vi "SCREEN_1.vi"(8 "error in (no error)":errorcluster, 11 "Main_Data_Flow":T1={"Hardware Setting"=path "", "Hardware"={"Monitor Primary 1"=1, "Monitor 2"=2, "Monitor 3"=3, "Scanner IP"="", "Scanner 2"="", "Scanner 3"="", "Printer IP"="", "Printer 2"="", "Printer 3"=""}, "SOP Path"=path "", "PNR Path"=path "", "PRN Data"=""}) -> (0 "error OUT":errorcluster)   [LabVIEW 2017]
doc: "Use this template to build a user interface event handler design pattern. Use this pattern for dialog boxes and other user interfaces. You also can create and execute user-defined events that the VI can handle the same way as user interface events."
uses:
  Controls/Main_Loop_Data_Flow.ctl
  Controls/PLC_DATA_READ.ctl
  Controls/PLC_DATA_WRITE.ctl
  Controls/AUTO_STATE_QUEUE.ctl
  Controls/Screen1_st.ctl
  <vilib>/Utility/error.llb/DialogType.ctl
  <userlib>/_OpenG.lib/array/array.llb/Sort 1D Array (I32)__ogtk.vi
  <vilib>/Utility/config.llb/Read Key (U32).vi
  <vilib>/Utility/config.llb/NI_LVConfig.lvlib
panel:
  out "Scanner Status":bool
  out "Scanned data":string
  out "Stop scanner":bool
  out "date/time string":string
  out "Varient Running":string
  out "Error Status in PLC Loop":errorcluster
  out "DATE/TIME":string
  out "Machine Name":string
  out "Weight":i32 format="%.0f gm"
  out "Cycle Result":bool
  out "Dispaly No.":string
  out "PLC to Labview Data":i32[](array[numeric])
  out "Cycle Status":string
  out "Scan Code":string
  out "sop picture":picture
  in  "Close":bool
  # "Resolution: 1920 x 1080 pixels"
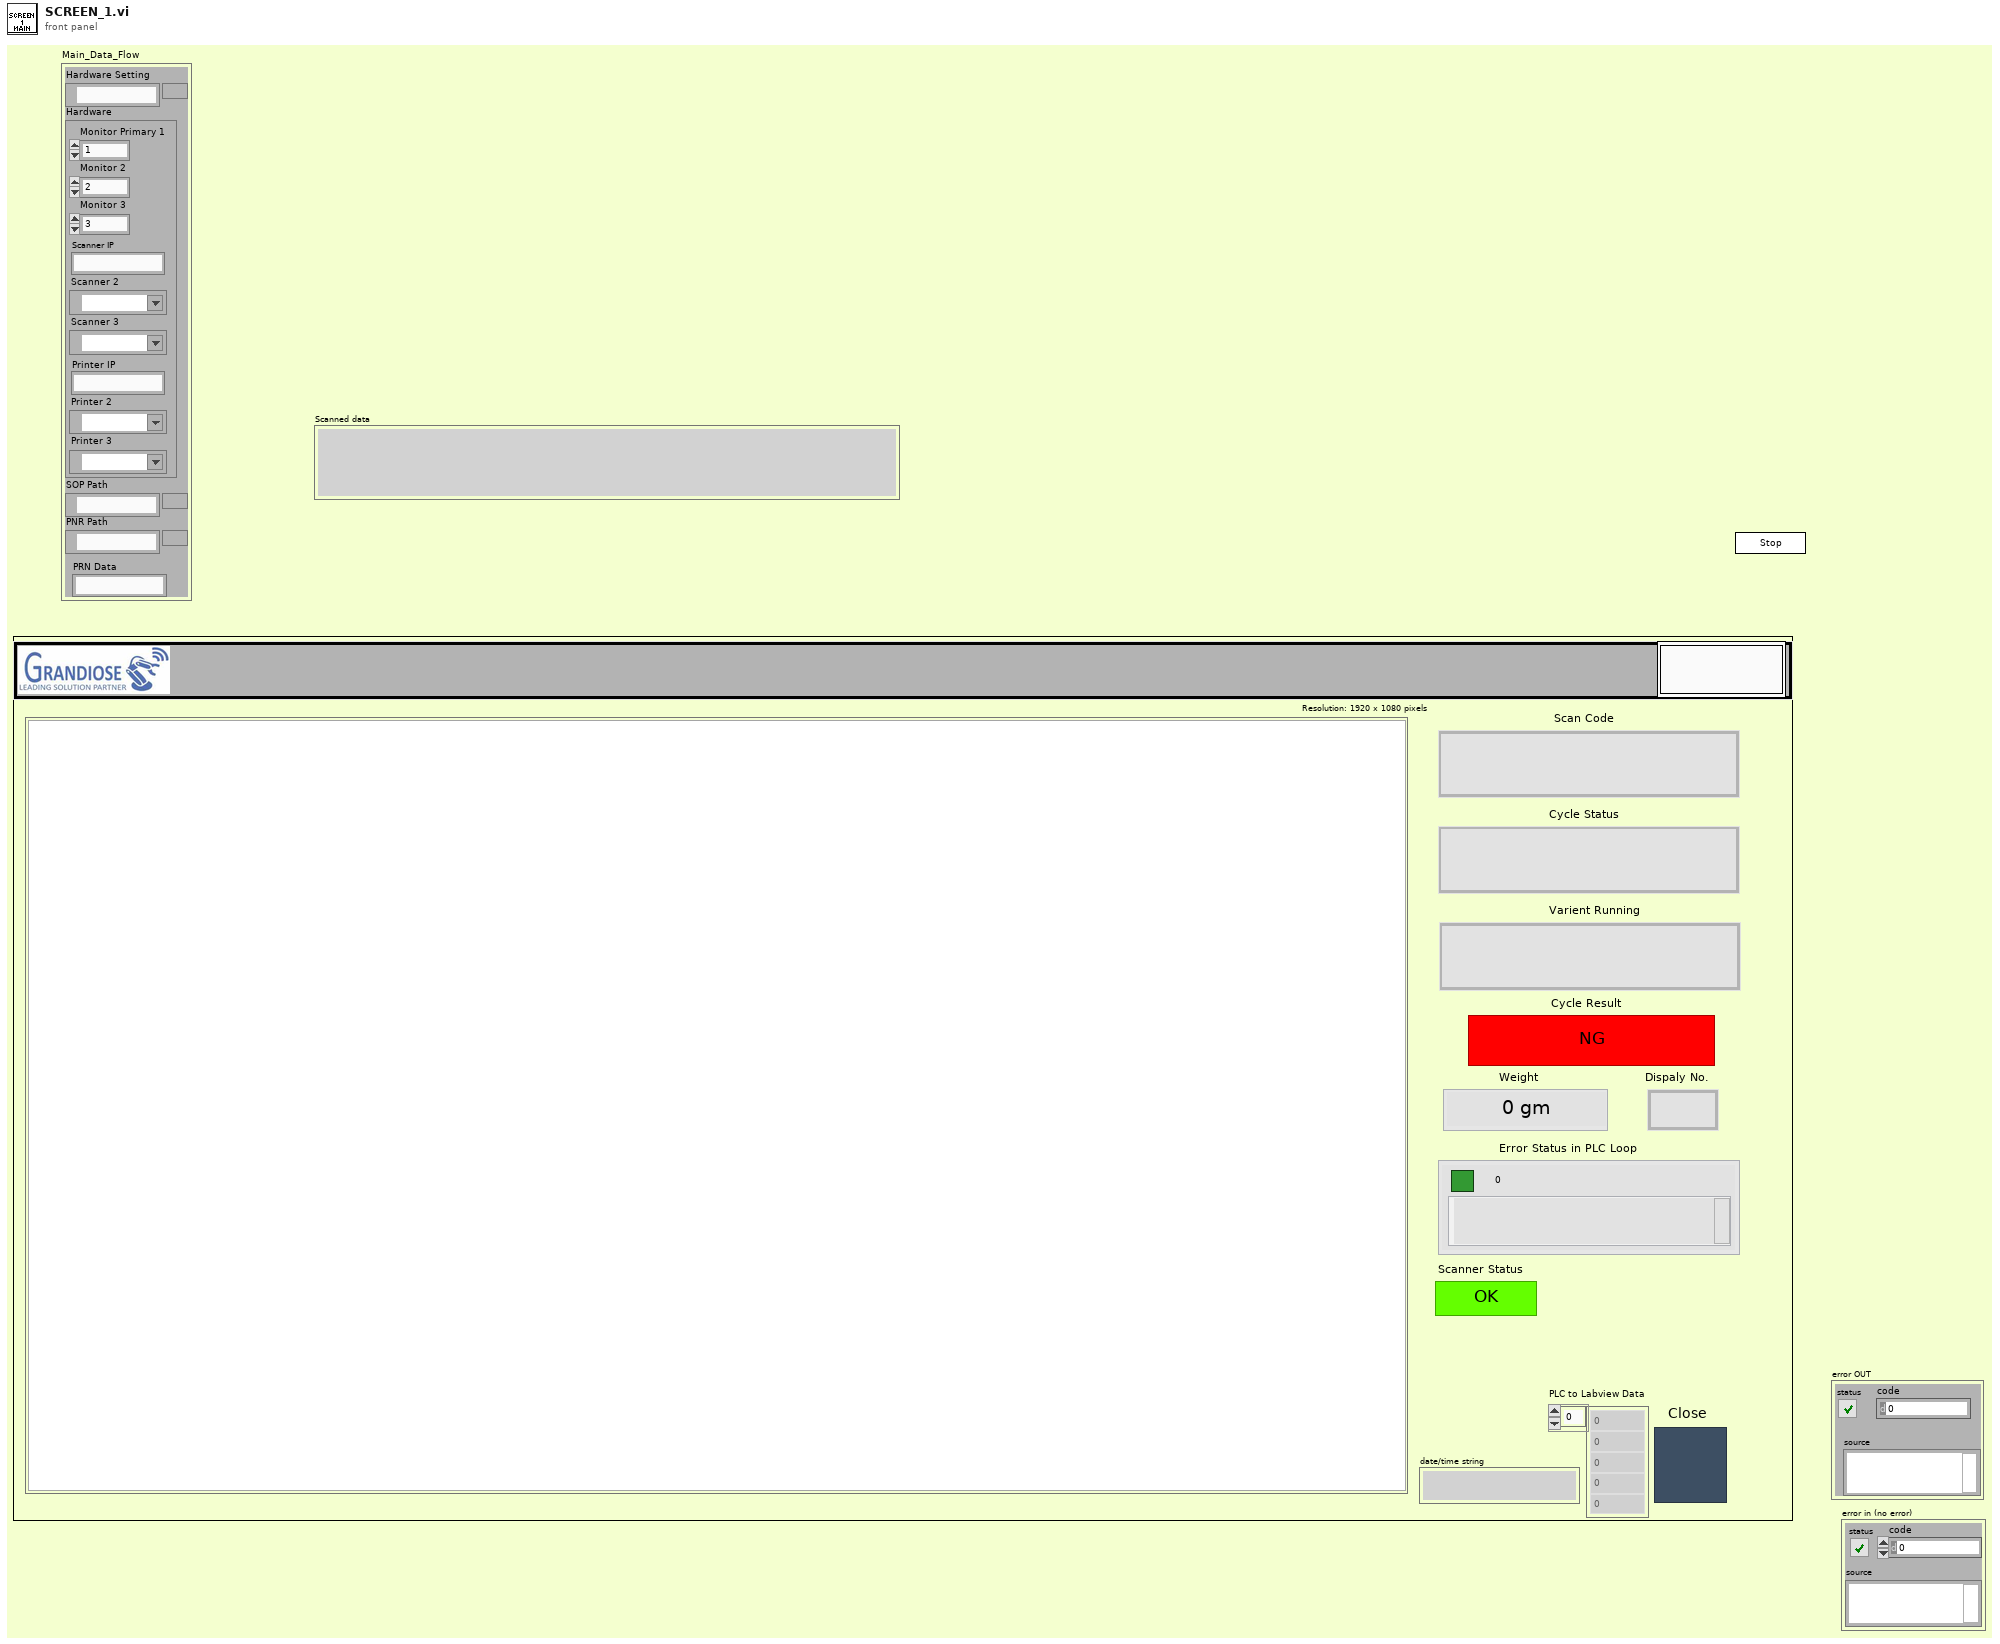
[diagram p1: front panel]
types:
  T1 = typedef "Main_Loop_Data_Flow.ctl" = cluster{"Hardware Setting":path, "Hardware":cluster{"Monitor Primary 1":u16, "Monitor 2":u16, "Monitor 3":u16, "Scanner IP":string, "Scanner 2":refnum<visa-resource-name>, "Scanner 3":refnum<visa-resource-name>, "Printer IP":string, "Printer 2":refnum<visa-resource-name>, "Printer 3":refnum<visa-resource-name>}, "SOP Path":path, "PNR Path":path, "PRN Data":string}
  T2 = typedef "AUTO_STATE_QUEUE.ctl" = enum16{"CREATE Q", "EN Q", "DE Q", "CLOSE Q"}
  T3 = typedef "PLC_DATA_READ.ctl" = cluster{"PLC to Labview Data":i32[], "Error Status in PLC Loop":errorcluster}
  T4 = cluster{"notifier out":refnum<notifier>, "SOP Path":path, "All Files SOP":path[], "PLC RCV data":T3, "Varient No.":u32[], "Varient name":string[], "Scanner IP":string, "Printer IP":string, "Printer ref":refnum<k5>, "PRN Data":string, "queue out":refnum<queue>}
  T5 = typedef "DialogType.ctl" = u16
  T6 = typedef "Screen1_st.ctl" = enum16{"Int", "Int2", "Wait", "Cluster_Update", "Cycle_Cmplt", "Varient_Updated", "Print_Code", "Error_Handling", "Exit"}
  T7 = typedef "imagedata.ctl" = cluster{"image type":i32, "image depth":i32, "image":u8[], "mask":u8[], "colors":u32[], "Rectangle":cluster{"left":i16, "top":i16, "right":i16, "bottom":i16}}
  T8 = typedef "PLC_DATA_WRITE.ctl" = cluster{"Register to write":u16, "Labview to PLC Data":u16}
  T9 = enum32{"invalid app kind", "Development System", "Run Time System", "Student Edition", "Embedded LabVIEW", "Evaluation", "Custom"}
  T10 = typedef "NI_LVConfig.lvlib/Config Data RefNum.ctl" = refnum<k1>
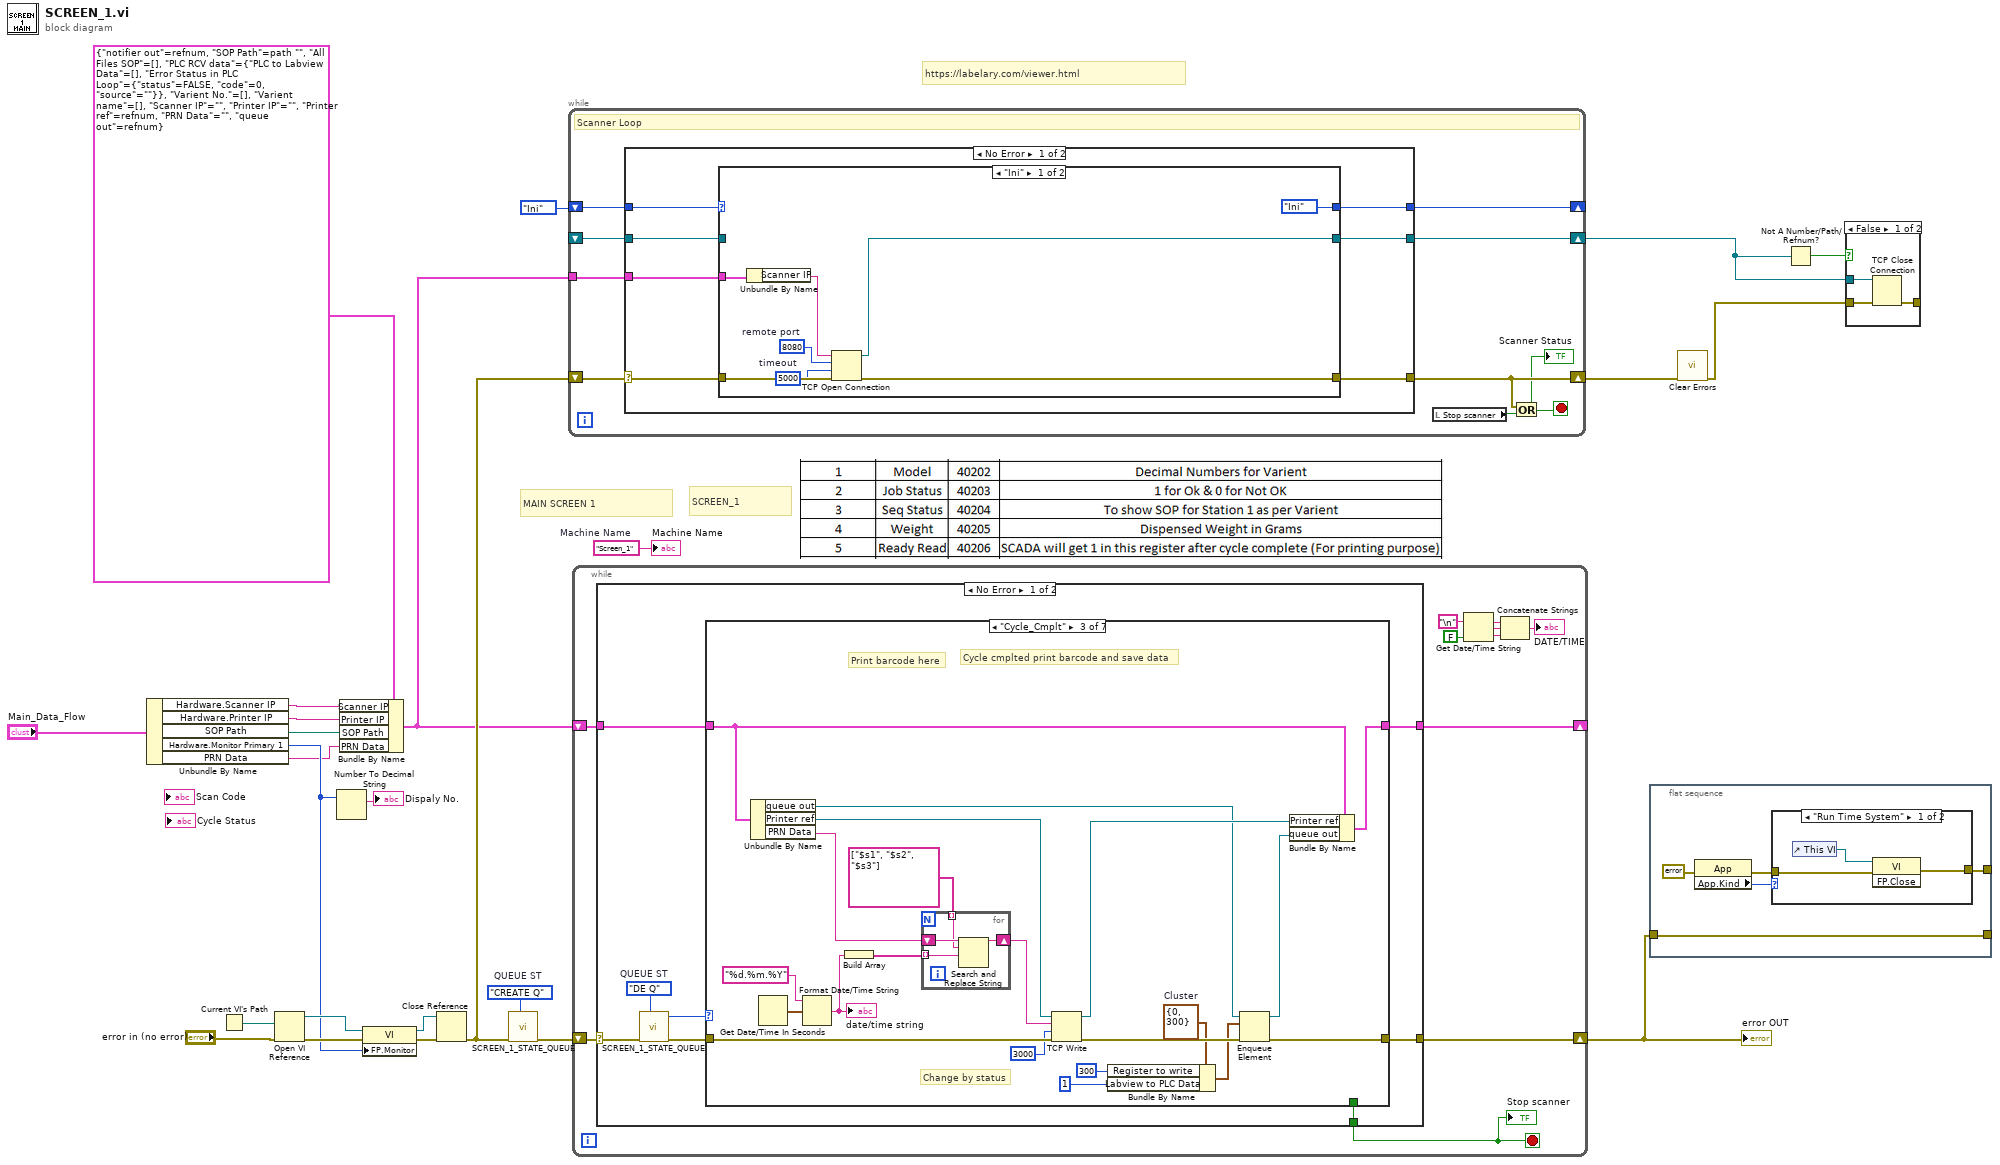
[diagram p0: block diagram]
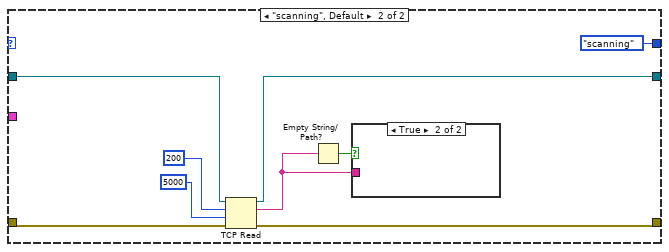
[diagram p3: hidden frame]
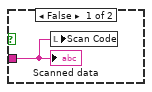
[diagram p4: hidden frame]
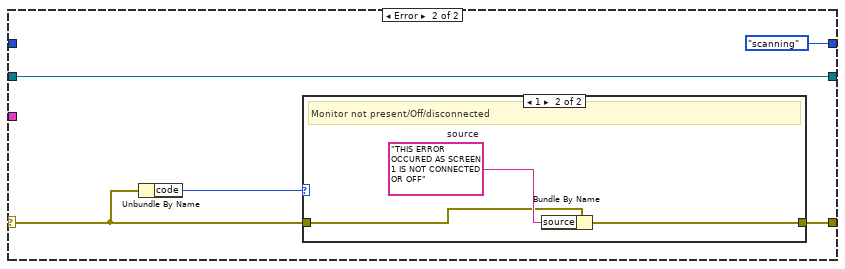
[diagram p5: hidden frame]
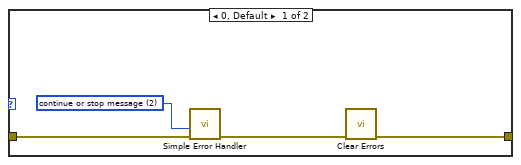
[diagram p6: hidden frame]
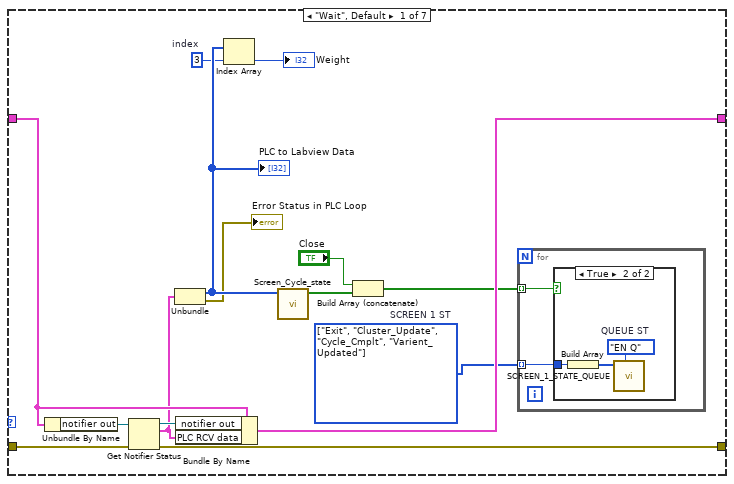
[diagram p8: hidden frame]
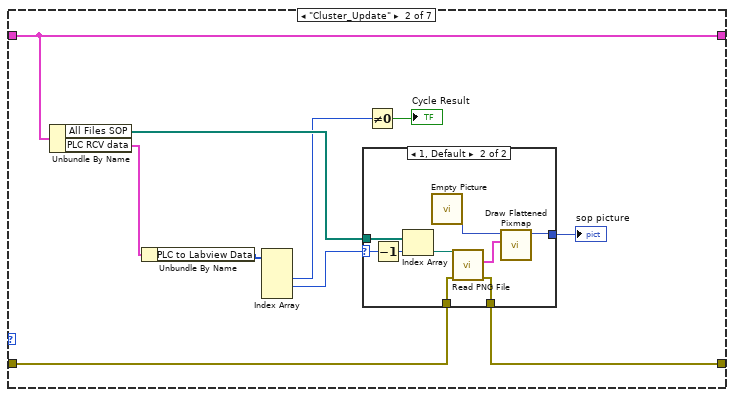
[diagram p10: hidden frame]
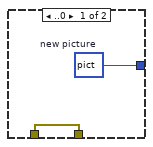
[diagram p11: hidden frame]
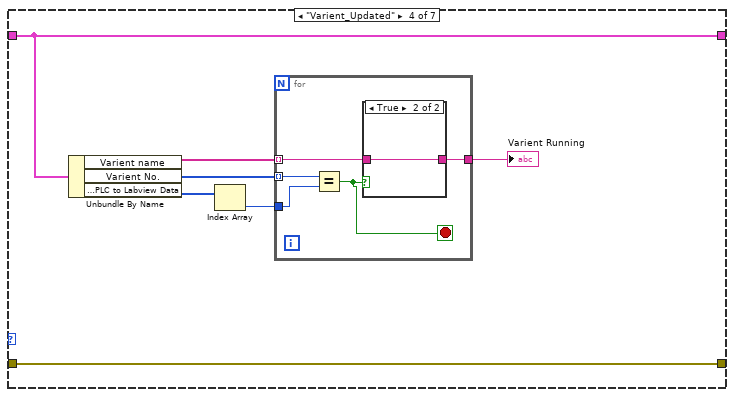
[diagram p12: hidden frame]
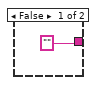
[diagram p13: hidden frame]
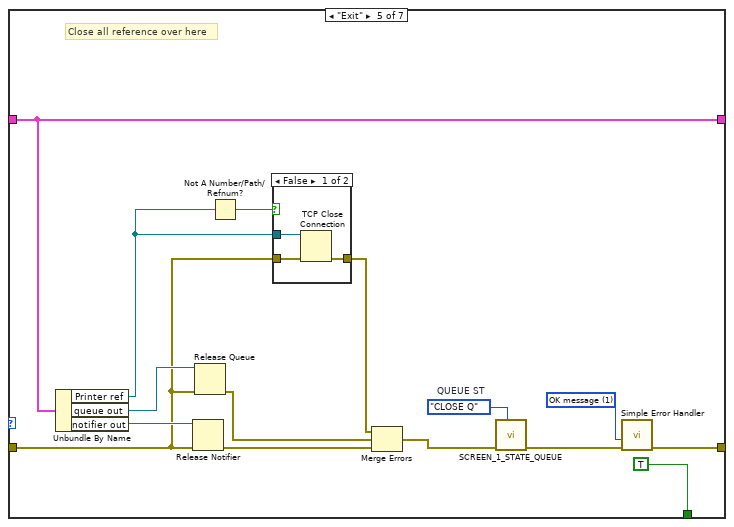
[diagram p14: hidden frame]
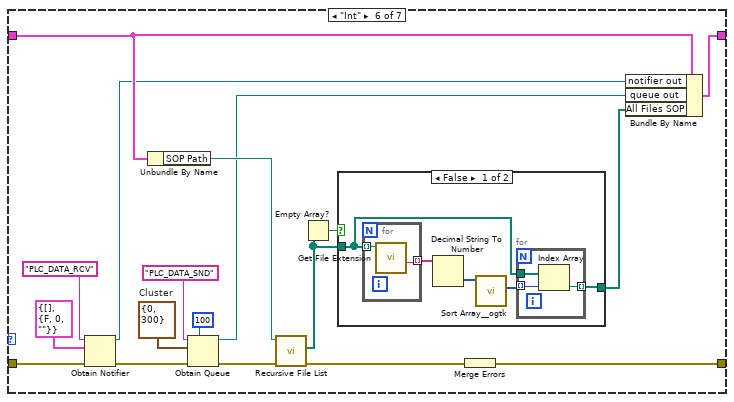
[diagram p16: hidden frame]
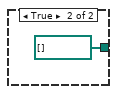
[diagram p17: hidden frame]
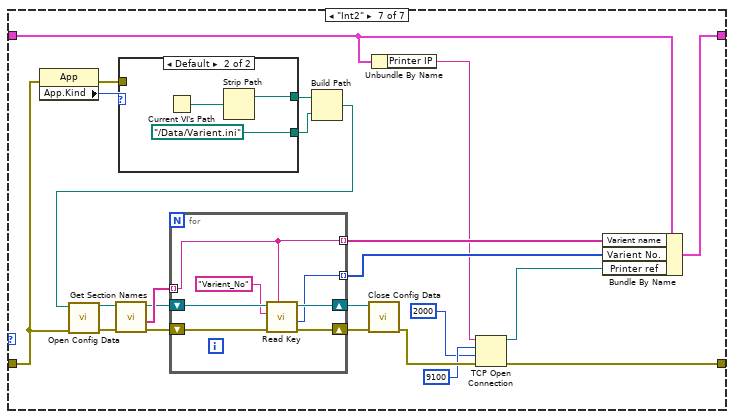
[diagram p18: hidden frame]
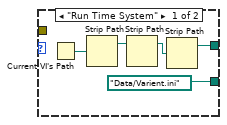
[diagram p19: hidden frame]
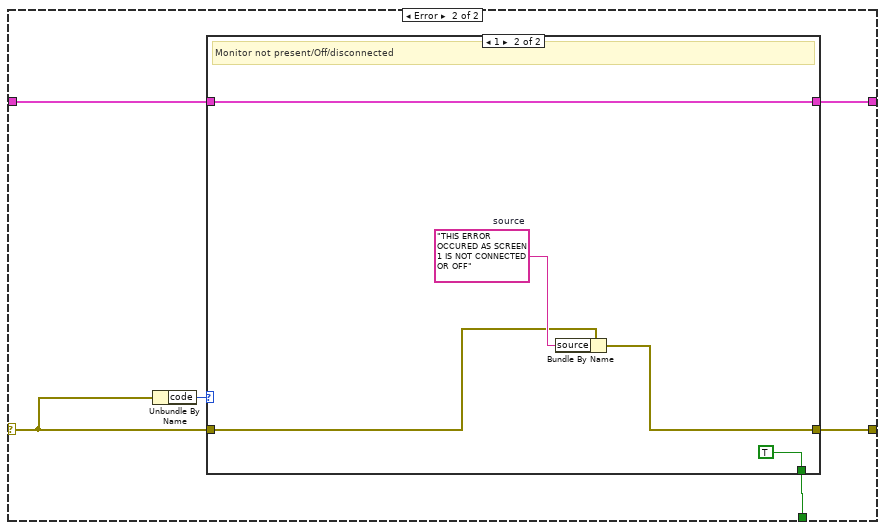
[diagram p20: hidden frame]
diagram:
  w10 = AUTO_STATE_QUEUE."CREATE Q"  # QUEUE ST
  w19 = "Screen_1"  # Machine Name
  # "https://labelary.com/viewer.html"
  # "MAIN SCREEN 1"
  # "SCREEN_1"
  n1 = Unbundle By Name("Main_Data_Flow") -> ("Hardware.Scanner IP"=w15:string, "Hardware.Printer IP"=w16:string, "SOP Path"=w9:path, "Hardware.Monitor Primary 1"=w12:u16, "PRN Data"=w8:string)
  n2 = Current VI's Path() -> (path=w25:path)
  n3 = Open VI Reference(vi path=w25, error in (no error)="error in (no error)") -> (vi reference=w21:refnum<vi>, error out=w22:errorcluster)  [unwired: 4 in]
  n4 = Number To Decimal String(number=w12) -> (decimal integer string=→"Dispaly No.":string)  [unwired: 1 in]
  n5 = Bundle By Name(cluster=T4 {"notifier out"=refnum, "SOP Path"=path "", "All Files SOP"=[], "PLC RCV data"={"PLC to Labview Data"=[], "Error Status in PLC Loop"={"status"=FALSE, "code"=0, "source"=""}}, "Varient No."=[], "Varient name"=[], "Scanner IP"="", "Printer IP"="", "Printer ref"=refnum, "PRN Data"="", "queue out"=refnum}, "Scanner IP"=w15, "Printer IP"=w16, "SOP Path"=w9, "PRN Data"=w8) -> (w5:T4)
  n6 = property class="VI"(reference=w21, error in=w22, "FP.Monitor"=w12) -> (reference out=w24:refnum<vi>, error out=w23:errorcluster)
  n7 = Close Reference(reference=w24, error in (no error)=w23) -> (error out=w7:errorcluster)
  n8 = call "SCREEN_1_STATE_QUEUE.vi"("QUEUE ST"=w10, "error in"=w7) -> ("error OUT"=w11:errorcluster)  [unwired: 8 in, 1 out]
  n9 = while {
    shift-right: [w32] -> w4
    shift-left: w7 -> [w34]
    shift-right: [w30] -> _
    shift-left: enum16{"Ini", "scanning", "Close"}."Ini" -> [w31]
    tunnel: w5 -> [w29]
    shift-right: [w28] -> w1
    shift-left: _ -> [w27]
    stop <- w26 stop-if-true
    # "Scanner Loop"
    n10 = case shown="No Error" w34 {
      selector: w34 -> [w41 w63]
      tunnel: [w40 w62] -> w32
      tunnel: w31 -> [w39 _]
      tunnel: [w38 enum16{"Ini", "scanning", "Close"}."scanning"] -> w30
      tunnel: w29 -> [w37 _]
      tunnel: [w36 w60] -> w28
      tunnel: w27 -> [w35 w60]
      frame No Error {
        n11 = case shown="\"Ini\"" w39 {
          tunnel: w41 -> [w47 w53]
          tunnel: [w46 w52] -> w40
          tunnel: [enum16{"Ini", "scanning", "Close"}."Ini" enum16{"Ini", "scanning", "Close"}."scanning"] -> w38
          tunnel: w37 -> [w48 _]
          tunnel: [w42 w50] -> w36
          tunnel: w35 -> [_ w51]
          frame "Ini" {
            w43 = 5000  # timeout
            w44 = u16 8080  # remote port
            n12 = Unbundle By Name(w48) -> ("Scanner IP"=w45:string)
            n13 = TCP Open Connection(address=w45, remote port or service name=w44, timeout ms (60000)=w43, error in (no error)=w47) -> (connection ID=w42:refnum<k5>, error out=w46:errorcluster)  [unwired: 1 in]
          }
          frame "scanning", Default {
            n14 = TCP Read(connection ID=w51, bytes to read=200, error in (no error)=w53, 9:5000 ("timeout ms (25000)")) -> (connection ID out=w50:refnum<k5>, data out=w56:string, error out=w52:errorcluster)  [unwired: 1 in]
            n15 = Empty String/Path?(string/path=w56) -> (empty?=w57:bool)
            n16 = case shown="True" w57 {
              tunnel: w56 -> [w59 _]
              frame False {
                n17 = local write "Scan Code"(w59) -> ()
                "Scanned data" <- w59
              }
              frame True {
              }
            }
          }
        }
      }
      frame Error {
        n18 = Unbundle By Name(w63) -> ("code"=w64:i32)
        n19 = case shown="1" w64 {
          tunnel: w63 -> [w68 w70]
          tunnel: [w66 w69] -> w62
          frame 0, Default {
            w65 = T5 2 items=["no dialog", "OK message", "continue or stop message", "OK message + warnings", "continue/stop + warnings"] ("type of dialog (OK msg:1)")
            n20 = call <vilib>:"Simple Error Handler.vi"("type of dialog (OK msg:1)"=w65, "error in (no error)"=w68) -> ("error out"=w67:errorcluster)  [unwired: 3 in, 4 out]
            n21 = call <vilib>:"Clear Errors.vi"("error in (no error)"=w67) -> ("error out"=w66:errorcluster)  [unwired: 5 in, 1 out]
          }
          frame 1 {
            w71 = "THIS ERROR OCCURED AS SCREEN 1 IS NOT CONNECTED OR OFF"  # source
            # "Monitor not present/Off/disconnected"
            n22 = Bundle By Name(cluster=w70, "source"=w71) -> (w69:errorcluster)
          }
        }
      }
    }
    n23 = local read "Stop scanner"() -> (w33:bool)
    n24 = Or(x=w32, y=w33) -> (x .or. y?=w26:bool)
    "Scanner Status" <- w26
  }
  n25 = while {
    shift-right: [w81] -> w14
    shift-left: w11 -> [w80]
    shift-right: [w78] -> _
    shift-left: w5 -> [w79]
    stop <- w72 stop-if-true
    n26 = case shown="No Error" w80 {
      selector: w80 -> [w86 w259]
      tunnel: [w82 w260] -> w72
      tunnel: [w89 w261] -> w81
      tunnel: w79 -> [w88 w257]
      tunnel: [w87 w256] -> w78
      frame No Error {
        w84 = AUTO_STATE_QUEUE."DE Q"  # QUEUE ST
        n27 = call "SCREEN_1_STATE_QUEUE.vi"("QUEUE ST"=w84, "error in"=w86) -> ("error OUT"=w85:errorcluster, "SCREEN 1"=w83:T6)  [unwired: 8 in]
        n28 = case shown="\"Cycle_Cmplt\"" w83 {
          tunnel: w85 -> [w104 w117 w151 w162 w172 w201 w229]
          tunnel: [w103 w116 w137 w162 w179 w206 w224] -> w89
          tunnel: w88 -> [w99 w119 w148 w161 w184 w205 w223]
          tunnel: [w100 w119 w147 w161 w184 w204 w228] -> w87
          tunnel: [_ _ _ _ TRUE _ _] -> w82
          frame "Wait", Default {
            w92 = 3  # index
            w95 = T6[] [enum."Exit", enum."Cluster_Update", enum."Cycle_Cmplt", enum."Varient_Updated"] items=["Int", "Int2", "Wait", "Cluster_Update", "Cycle_Cmplt", "Varient_Updated", "Print_Code", "Error_Handling", "Exit"]  # SCREEN 1 ST
            n29 = Unbundle By Name(w99) -> ("notifier out"=w102:refnum<notifier>)
            n30 = Get Notifier Status(notifier=w102, error in (no error)=w104) -> (notifier out=w101:refnum<notifier>, current notification=w91:T3, error out=w103:errorcluster)  [unwired: 2 out]
            n31 = Unbundle(w91) -> ("PLC to Labview Data"=w93:i32[], "Error Status in PLC Loop"=→"Error Status in PLC Loop":errorcluster)
            "PLC to Labview Data" <- w93
            n32 = Bundle By Name(cluster=w99, "notifier out"=w101, "PLC RCV data"=w91) -> (w100:T4)
            n33 = Index Array(array=w93, index=w92) -> (element=→"Weight":i32)
            n34 = call "Screen_Cycle_state.vi"("PLC to Labview Data"=w93) -> ("Cyc St"=w97:bool[])  [unwired: 10 in]
            n35 = Build Array (concatenate)("Close", w97) -> (w96:bool[])
            n36 = for {
              tunnel: w96 -> [w106] mode=indexing
              tunnel: w95 -> [w105] mode=indexing
              n37 = case shown="True" w106 {
                tunnel: w105 -> [_ w108]
                frame False {
                }
                frame True {
                  w109 = AUTO_STATE_QUEUE."EN Q"  # QUEUE ST
                  n38 = Build Array(w108) -> (w107:T6[])
                  n39 = call "SCREEN_1_STATE_QUEUE.vi"("QUEUE ST"=w109, "SCREEN 1 ST"=w107) -> ()  [unwired: 8 in, 2 out]
                }
              }
            }
          }
          frame "Cluster_Update" {
            n40 = Unbundle By Name(w119) -> ("All Files SOP"=w118:path[], "PLC RCV data"=w115:T3)
            n41 = Unbundle By Name(w115) -> ("PLC to Labview Data"=w114:i32[])
            n42 = Index Array(array=w114) -> (element #2=w111:i32, element #3=w113:i32)  [unwired: 4 in, 2 out]
            n43 = case shown="1, Default" w113 {
              selector: w113 -> [_ w124]
              tunnel: w118 -> [_ w127]
              tunnel: w117 -> [w121 w126]
              tunnel: [w121 w125] -> w116
              tunnel: [w120 w122] -> w110
              frame ..0 {
                w120 = picture data[5B]  # new picture
              }
              frame 1, Default {
                n44 = Decrement(x=w124) -> (x-1=w123:i32)
                n45 = Index Array(array=w127, index=w123) -> (element=w128:path)
                n46 = call "Empty Picture"() -> ("empty picture"=w129:picture)
                n47 = call <vilib>:"Read PNG File.vi"("error in (no error)"=w126, "path to PNG file"=w128) -> ("error out"=w125:errorcluster, "image data"=w130:T7)  [unwired: 7 in, 1 out]
                n48 = call <vilib>:"Draw Flattened Pixmap.vi"("image data"=w130, "picture"=w129) -> ("new picture"=w122:picture)  [unwired: 7 in]
              }
            }
            "sop picture" <- w110
            n49 = Not Equal To 0?(x=w111) -> (x != 0?=→"Cycle Result":bool)
          }
          frame "Cycle_Cmplt" {
            w134 = T8 {"Register to write"=0, "Labview to PLC Data"=300}  # Cluster
            # "Change by status"
            # "Print barcode here"
            # "Cycle cmplted print barcode and save data"
            n50 = Unbundle By Name(w148) -> ("queue out"=w136:refnum<queue>, "Printer ref"=w149:refnum<k5>, "PRN Data"=w141:string)
            n51 = Get Date/Time In Seconds() -> (seconds since 1Jan1904=w144:timestamp)
            n52 = Format Date/Time String(time format string (%c)="%d.%m.%Y", seconds (now)=w144) -> (date/time string=w139:string)  [unwired: 1 in]
            "date/time string" <- w139
            n53 = Build Array(w139) -> (w138:string[])
            n54 = for {
              shift-right: [w155] -> w140
              shift-left: w141 -> [w154]
              tunnel: string[] ["$s1", "$s2", "$s3"] -> [w153] mode=indexing
              tunnel: w138 -> [w152] mode=indexing
              n55 = Search and Replace String(input string=w154, search string=w153, replace string=w152) -> (result string=w155:string)  [unwired: 5 in, 3 out]
            }
            n56 = TCP Write(connection ID=w149, data in=w140, error in (no error)=w151, 9:3000 ("timeout ms (25000)")) -> (connection ID out=w146:refnum<k5>, error out=w150:errorcluster)  [unwired: 1 out]
            n57 = Bundle By Name(cluster=w134, "Register to write"=u16 300 ("timeout ms (25000)"), "Labview to PLC Data"=u16 1 ("timeout ms (25000)")) -> (w133:T8)
            n58 = Enqueue Element(queue=w136, element=w133, error in (no error)=w150) -> (queue out=w135:refnum<queue>, error out=w137:errorcluster)  [unwired: 1 in, 1 out]
            n59 = Bundle By Name(cluster=w148, "Printer ref"=w146, "queue out"=w135) -> (w147:T4)
          }
          frame "Varient_Updated" {
            n60 = Unbundle By Name(w161) -> ("Varient name"=w157:string[], "Varient No."=w159:u32[], "PLC RCV data.PLC to Labview Data"=w160:i32[])
            n61 = Index Array(array=w160) -> (element=w158:i32)  [unwired: 1 in]
            n62 = for {
              tunnel: w159 -> [w167] mode=indexing
              tunnel: w158 -> [w166]
              tunnel: [w165] -> w156
              tunnel: w157 -> [w164] mode=indexing
              stop <- w163 stop-if-true
              n63 = Equal?(x=w167, y=w166) -> (x = y?=w163:bool)
              n64 = case shown="True" w163 {
                tunnel: ["" w169] -> w165
                tunnel: w164 -> [_ w169]
                frame False {
                }
                frame True {
                }
              }
            }
            "Varient Running" <- w156
          }
          frame "Exit" {
            w178 = T5 1 items=["no dialog", "OK message", "continue or stop message", "OK message + warnings", "continue/stop + warnings"] ("type of dialog (OK msg:1)")
            w181 = AUTO_STATE_QUEUE."CLOSE Q"  # QUEUE ST
            # "Close all reference over here"
            n65 = Unbundle By Name(w184) -> ("Printer ref"=w174:refnum<k5>, "queue out"=w173:refnum<queue>, "notifier out"=w183:refnum<notifier>)
            n66 = Release Notifier(notifier=w183, error in (no error)=w172) -> (error out=w175:errorcluster)  [unwired: 1 in, 2 out]
            n67 = Release Queue(queue=w173, error in (no error)=w172) -> (error out=w170:errorcluster)  [unwired: 1 in, 2 out]
            n68 = Not A Number/Path/Refnum?(number/path/refnum=w174) -> (NaN/Path/Refnum?=w177:bool)
            n69 = case shown="False" w177 {
              tunnel: w172 -> [w187 w188]
              tunnel: w174 -> [w186 _]
              tunnel: [w185 w188] -> w171
              frame False {
                n70 = TCP Close Connection(connection ID=w186, error in (no error)=w187) -> (error out=w185:errorcluster)  [unwired: 2 out]
              }
              frame True {
              }
            }
            n71 = Merge Errors(w171, w170, w175) -> (w176:errorcluster)
            n72 = call "SCREEN_1_STATE_QUEUE.vi"("QUEUE ST"=w181, "error in"=w176) -> ("error OUT"=w180:errorcluster)  [unwired: 8 in, 1 out]
            n73 = call <vilib>:"Simple Error Handler.vi"("type of dialog (OK msg:1)"=w178, "error in (no error)"=w180) -> ("error out"=w179:errorcluster)  [unwired: 3 in, 4 out]
          }
          frame "Int" {
            w194 = T8 {"Register to write"=0, "Labview to PLC Data"=300}  # Cluster
            n74 = Obtain Notifier(name (unnamed)="PLC_DATA_RCV", notification data type=T3 {"PLC to Labview Data"=[], "Error Status in PLC Loop"={"status"=FALSE, "code"=0, "source"=""}}, error in (no error)=w201) -> (notifier out=w198:refnum<notifier>, error out=w192:errorcluster)  [unwired: 1 in, 1 out]
            n75 = Unbundle By Name(w205) -> ("SOP Path"=w200:path)
            n76 = Obtain Queue(max queue size (-1, unlimited)=100, name (unnamed)="PLC_DATA_SND", element data type=w194, error in (no error)=w192) -> (queue out=w189:refnum<queue>, error out=w191:errorcluster)  [unwired: 1 in, 1 out]
            n77 = call <vilib>:"Recursive File List.vi"("error in (no error)"=w191, "Folder Path"=w200) -> ("error out"=w199:errorcluster, "All Files in Dir"=w196:path[])  [unwired: 5 in, 3 out]
            n78 = Empty Array?(array=w196) -> (empty?=w197:bool)
            n79 = case shown="False" w197 {
              tunnel: w196 -> [w210 _]
              tunnel: [w207 path[] []] -> w190
              frame False {
                n80 = for {
                  tunnel: [w216] -> w209 mode=indexing
                  tunnel: w210 -> [w215] mode=indexing
                  n81 = call <vilib>:"Get File Extension.vi"("file"=w215) -> ("filename without extension"=w216:string)  [unwired: 6 in, 4 out]
                }
                n82 = Decimal String To Number(string=w209) -> (number=w208:i32[])  [unwired: 2 in, 1 out]
                n83 = call-poly <userlib>:"Sort Array__ogtk.vi"("Array in"=w208) -> ("Sorted Pointers"=w211:i32[])  [unwired: 9 in, 1 out]
                n84 = for {
                  tunnel: w211 -> [w214] mode=indexing
                  tunnel: w210 -> [w213]
                  tunnel: [w212] -> w207 mode=indexing
                  n85 = Index Array(array=w213, index=w214) -> (element=w212:path)
                }
              }
              frame True {
              }
            }
            n86 = Merge Errors(w199) -> (w206:errorcluster)
            n87 = Bundle By Name(cluster=w205, "notifier out"=w198, "queue out"=w189, "All Files SOP"=w190) -> (w204:T4)
          }
          frame "Int2" {
            n88 = property class="App"(error in=w229) -> (error out=w239:errorcluster, "App.Kind"=w237:T9)  [unwired: 1 in, 1 out]
            n89 = case shown="Default" w237 {
              tunnel: [path "Data/Varient.ini" ("path") path "../Data/Varient.ini" ("path")] -> w238
              tunnel: [w248 w253] -> w240
              tunnel: w239 -> [_ _]
              frame "Run Time System" {
                n90 = Current VI's Path() -> (path=w251:path)
                n91 = Strip Path(path=w251) -> (stripped path=w250:path)  [unwired: 1 out]
                n92 = Strip Path(path=w250) -> (stripped path=w249:path)  [unwired: 1 out]
                n93 = Strip Path(path=w249) -> (stripped path=w248:path)  [unwired: 1 out]
              }
              frame Default {
                n94 = Current VI's Path() -> (path=w254:path)
                n95 = Strip Path(path=w254) -> (stripped path=w253:path)  [unwired: 1 out]
              }
            }
            n96 = Build Path(base path=w240, name or relative path=w238) -> (appended path=w221:path)
            n97 = call <vilib>:"Open Config Data.vi"("error in (no error)"=w229, "configuration file path"=w221) -> ("error out"=w236:errorcluster, "refnum"=w235:T10)  [unwired: 7 in, 1 out]
            n98 = call <vilib>:"Get Section Names.vi"("error in (no error)"=w236, "refnum"=w235) -> ("error out"=w230:errorcluster, "section names"=w232:string[], "refnum out"=w231:T10)  [unwired: 7 in]
            n99 = for {
              shift-right: [w244] -> w233
              shift-left: w230 -> [w245]
              tunnel: w232 -> [w241] mode=indexing
              tunnel: [w242] -> w226 mode=indexing
              tunnel: [w241] -> w227 mode=indexing
              shift-right: [w246] -> w234
              shift-left: w231 -> [w247]
              n100 = call-poly <vilib>:"Read Key.vi"("section"=w241, "error in (no error)"=w245, "key"="Varient_No", "refnum"=w247) -> ("error out"=w244:errorcluster, "value"=w242:u32, "refnum out"=w246:T10)  [unwired: 4 in, 1 out]
            }
            n101 = call <vilib>:"Close Config Data.vi"("error in (no error)"=w233, "refnum"=w234) -> ("error out"=w225:errorcluster)  [unwired: 8 in, 1 out]
            n102 = Unbundle By Name(w223) -> ("Printer IP"=w222:string)
            n103 = TCP Open Connection(address=w222, remote port or service name=u16 9100, timeout ms (60000)=2000, error in (no error)=w225) -> (connection ID=w220:refnum<k5>, error out=w224:errorcluster)  [unwired: 1 in]
            n104 = Bundle By Name(cluster=w223, "Varient name"=w227, "Varient No."=w226, "Printer ref"=w220) -> (w228:T4)
          }
        }
      }
      frame Error {
        n105 = Unbundle By Name(w259) -> ("code"=w258:i32)
        n106 = case shown="1" w258 {
          tunnel: w259 -> [w266 w269]
          tunnel: [w263 w268] -> w261
          tunnel: [_ TRUE] -> w260
          tunnel: w257 -> [w265 w267]
          tunnel: [w265 w267] -> w256
          frame 0, Default {
            w262 = T5 2 items=["no dialog", "OK message", "continue or stop message", "OK message + warnings", "continue/stop + warnings"] ("type of dialog (OK msg:1)")
            n107 = call <vilib>:"Simple Error Handler.vi"("type of dialog (OK msg:1)"=w262, "error in (no error)"=w266) -> ("error out"=w264:errorcluster)  [unwired: 3 in, 4 out]
            n108 = call <vilib>:"Clear Errors.vi"("error in (no error)"=w264) -> ("error out"=w263:errorcluster)  [unwired: 5 in, 1 out]
          }
          frame 1 {
            w270 = "THIS ERROR OCCURED AS SCREEN 1 IS NOT CONNECTED OR OFF"  # source
            # "Monitor not present/Off/disconnected"
            n109 = Bundle By Name(cluster=w269, "source"=w270) -> (w268:errorcluster)
          }
        }
      }
    }
    "Stop scanner" <- w72
    n110 = Get Date/Time String(want seconds? (F)=FALSE) -> (date string=w76:string, time string=w77:string)  [unwired: 2 in]
    n111 = Concatenate Strings(w76, "\n", w77) -> (→"DATE/TIME":string)
  }
  "error OUT" <- w14
  n112 = flat-sequence {
    tunnel: [w273] -> _
    tunnel: [w272] -> _
    tunnel: w14 -> [w272]
    frame #0 {
      n113 = property class="App"(error in=errorcluster {"status"=FALSE, "code"=0, "source"=""} ("error in (no error)")) -> (error out=w275:errorcluster, "App.Kind"=w276:T9)  [unwired: 1 in, 1 out]
      n114 = case shown="\"Run Time System\"" w276 {
        tunnel: w275 -> [w278 w280]
        tunnel: [w277 w280] -> w273
        frame "Run Time System" {
          n115 = control-ref of="This VI"() -> (w279:refnum<vi>)
          n116 = invoke class="VI" method="FP.Close"(reference=w279, error in=w278) -> (error out=w277:errorcluster)  [unwired: 1 in, 2 out]
        }
        frame "Development System", Default {
        }
      }
    }
  }
  n117 = call <vilib>:"Clear Errors.vi"("error in (no error)"=w4) -> ("error out"=w2:errorcluster)  [unwired: 5 in, 1 out]
  n118 = Not A Number/Path/Refnum?(number/path/refnum=w1) -> (NaN/Path/Refnum?=w3:bool)
  n119 = case shown="False" w3 {
    tunnel: w2 -> [w283 w284]
    tunnel: w1 -> [w282 _]
    tunnel: [w281 w284] -> _
    frame False {
      n120 = TCP Close Connection(connection ID=w282, error in (no error)=w283) -> (error out=w281:errorcluster)  [unwired: 2 out]
    }
    frame True {
    }
  }
  "Machine Name" <- w19
